vi "Node - PXImc Write.vi"(8 "error in (no error)":errorcluster, 10 "Writer Data In":u8[](array[numeric]), 11 "Node Data In":T1) -> (0 "error out":errorcluster, 3 "Node Data Out":T1)   [LabVIEW 2016, in "PXImc Router.lvlib"]
uses:
  PXImc Router.lvlib
  Controls/Node Data.ctl
  Controls/Node/Node - PXImc Parameters.ctl
  Controls/Node/Node - Writer Data.ctl
  Controls/Node/Node Ch Properties.ctl
  Controls/Data Type.ctl
  Controls/Node/Node - Readers Data.ctl
  Controls/Node/Node - Reader Data.ctl
  <vilib>/pximc/Acquire Write Region (U8).vi
  <vilib>/pximc/nipximc.lvlib
  Engine/PXImc Custom Device Engine.lvlib
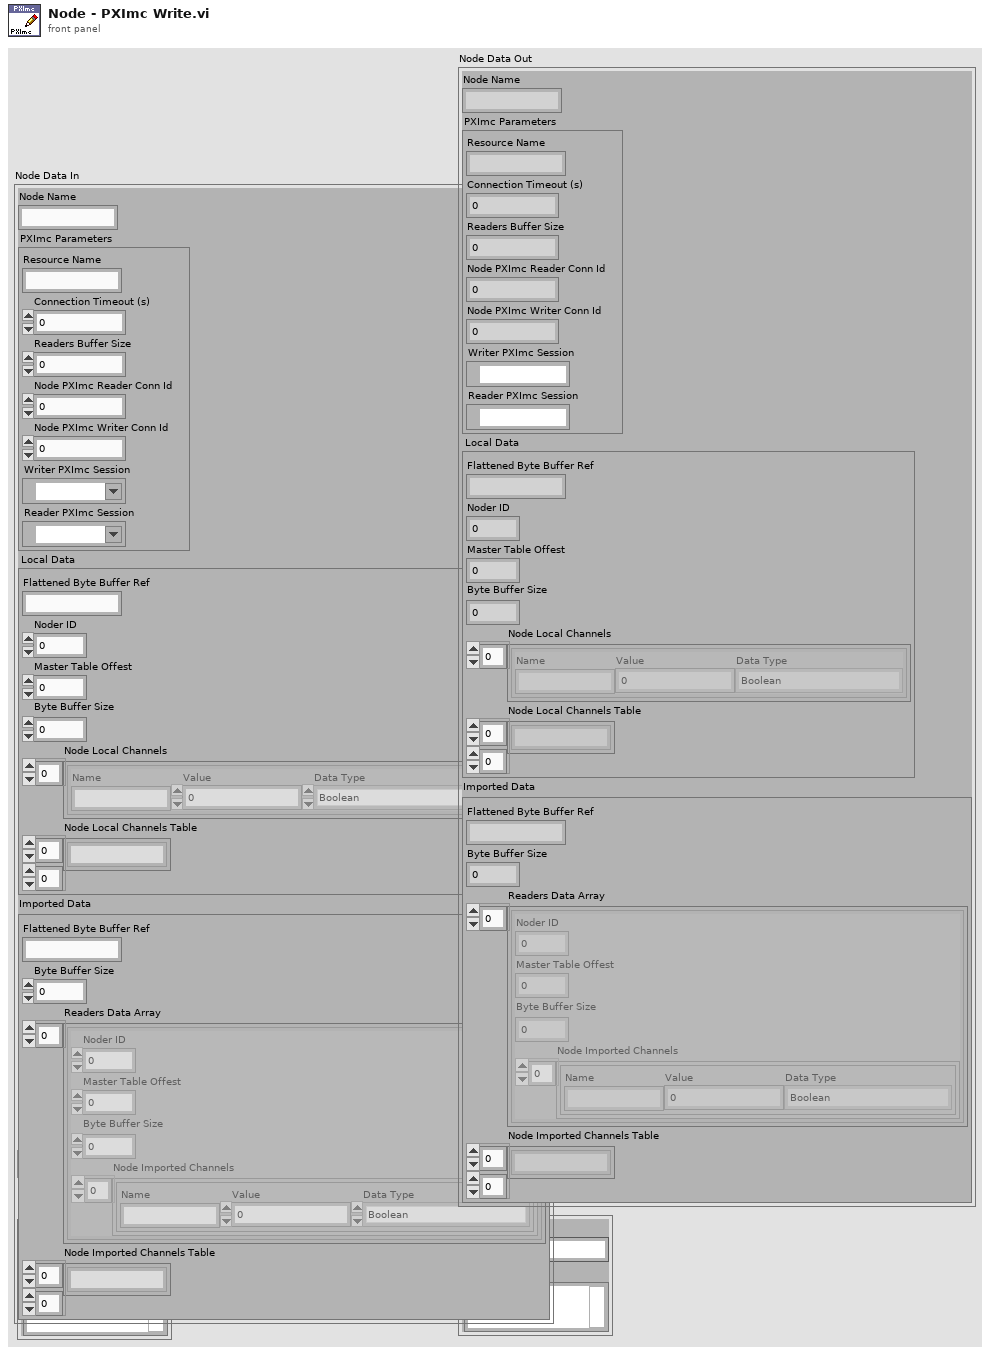
[diagram p1: front panel]
types:
  T1 = typedef "PXImc Router.lvlib/Node Data.ctl" = cluster{"Node Name":string, "PXImc Parameters":T2, "Local Data":T3, "Imported Data":T6}
  T2 = typedef "PXImc Router.lvlib/Node - PXImc Parameters.ctl" = cluster{"Resource Name":string, "Connection Timeout (s)":dbl, "Readers Buffer Size":u64, "Node PXImc Reader Conn Id":u16, "Node PXImc Writer Conn Id":u16, "Writer PXImc Session":refnum<k21>, "Reader PXImc Session":refnum<k21>}
  T3 = typedef "PXImc Router.lvlib/Node - Writer Data.ctl" = cluster{"Flattened Byte Buffer Ref":string, "Noder ID":u32, "Master Table Offest":u32, "Byte Buffer Size":u32, "Node Local Channels":T4[], "Node Local Channels Table":string[][]}
  T4 = typedef "PXImc Router.lvlib/Node Ch Properties.ctl" = cluster{"Name":string, "Value":dbl, "Data Type":T5}
  T5 = typedef "PXImc Router.lvlib/Data Type.ctl" = enum16{"Boolean", "SGL", "DBL", "I8", "I16", "I32", "I64", "U8", "U16", "U32", "U64"}
  T6 = typedef "PXImc Router.lvlib/Node - Readers Data.ctl" = cluster{"Flattened Byte Buffer Ref":string, "Byte Buffer Size":u64, "Readers Data Array":T7[], "Node Imported Channels Table":string[][]}
  T7 = typedef "PXImc Router.lvlib/Node - Reader Data.ctl" = cluster{"Noder ID":u32, "Master Table Offest":u32, "Byte Buffer Size":u64, "Node Imported Channels":T4[]}
  T8 = enum16{"Create File", "Log Message", "Log Error", "Log TimeStamp", "Close File"}
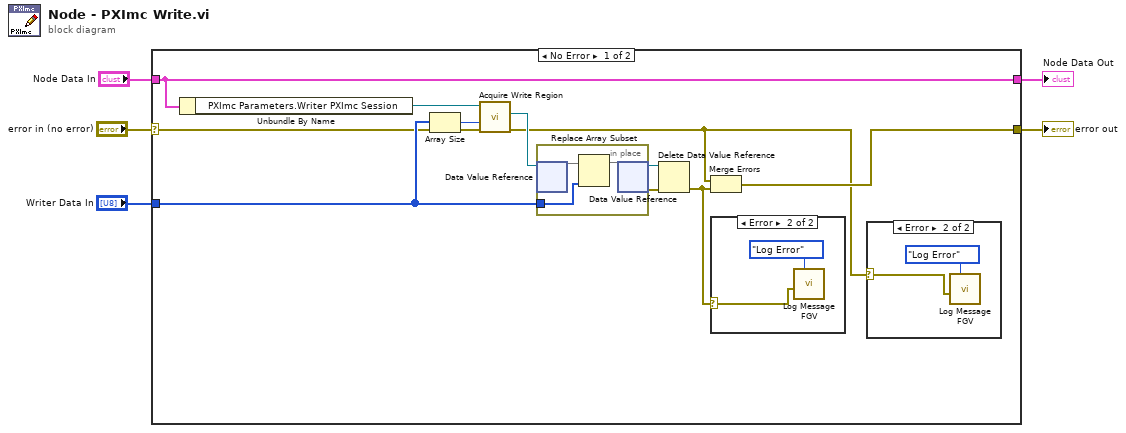
[diagram p0: block diagram]
diagram:
  n1 = case shown="No Error" "error in (no error)" {
    selector: "error in (no error)" -> [w9 w25]
    tunnel: "Writer Data In" -> [w16 _]
    tunnel: [w11 w25] -> w4
    tunnel: "Node Data In" -> [w8 w24]
    tunnel: [w8 w24] -> w1
    frame No Error {
      n2 = Unbundle By Name(w8) -> ("PXImc Parameters.Writer PXImc Session"=w10:refnum<k21>)
      n3 = Array Size(array=w16) -> (size(s)=w15:i32)
      n4 = call-poly <vilib>:"Acquire Write Region.vi"("error in (no error)"=w9, "number of elements"=w15, "session in"=w10) -> ("error out"=w6:errorcluster, "write region reference"=w14:refnum<data-value>)  [unwired: 5 in, 2 out]
      n5 = in-place {
        in-place-border: w16 -> [w21]
        n6 = in-place-dvr #1(w14) -> (w23:u8[])  [unwired: 1 out]
        n7 = Replace Array Subset(array=w23, new element=w21) -> (w22:u8[])  [unwired: 1 in]
        n8 = in-place-dvr #1(w22) -> (w13:refnum<data-value>, w12:errorcluster)
      }
      n9 = Delete Data Value Reference(data value reference=w13, error in=w12) -> (error out=w7:errorcluster)  [unwired: 1 out]
      n10 = Merge Errors(w6, w7) -> (w11:errorcluster)
      n11 = case shown="Error" w7 {
        selector: w7 -> [_ w19]
        frame No Error {
        }
        frame Error {
          n12 = call "Log Message FGV.vi"("FGV Cmd"=T8."Log Error", "Error In"=w19) -> ()  [unwired: 9 in, 1 out]
        }
      }
      n13 = case shown="Error" w6 {
        selector: w6 -> [_ w17]
        frame No Error {
        }
        frame Error {
          n14 = call "Log Message FGV.vi"("FGV Cmd"=T8."Log Error", "Error In"=w17) -> ()  [unwired: 9 in, 1 out]
        }
      }
    }
    frame Error {
    }
  }
  "error out" <- w4
  "Node Data Out" <- w1
